vi "getSubscriberInfo.vi"(0 "DeviceName":string="StagingAnalysis", 11 "error in (no error)":errorcluster) -> (4 "DeviceName out":string="StagingAnalysis", 6 "Devices":string[](array[string]), 8 "Alias":string[](array[string]), 10 "Variable header":string[](array[string]), 15 "error out":errorcluster)   [LabVIEW 2011]
panel:
  out "data":string[][](array[string])
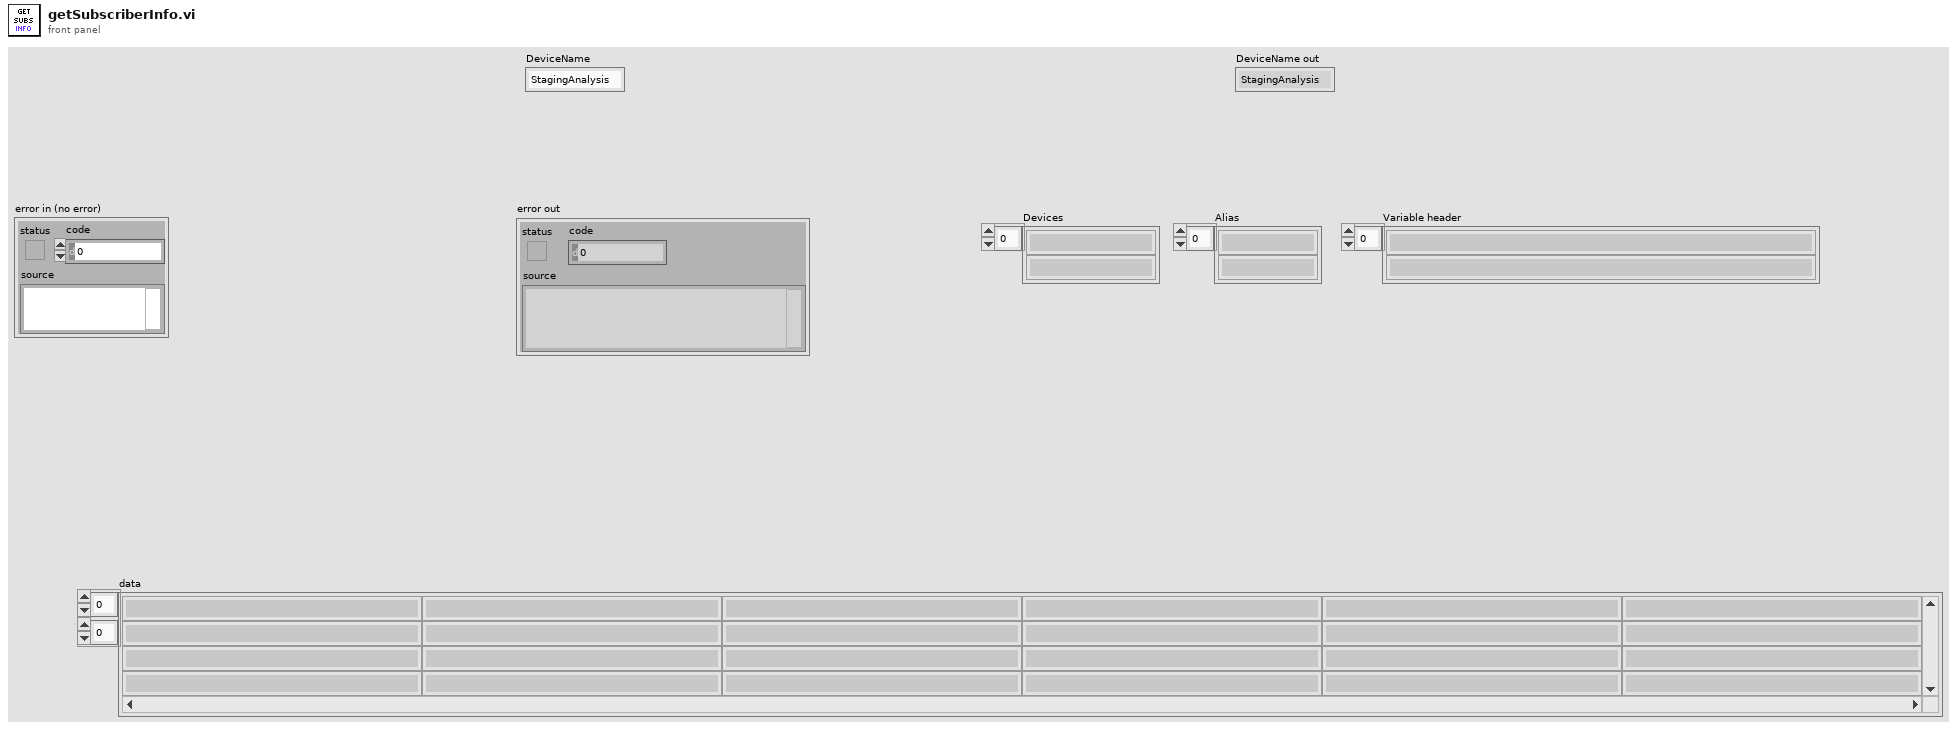
[diagram p1: front panel]
types:
  T1 = typedef "mysql_authentication.ctl" = cluster{"User":string, "Password":string, "Database":string}
  T2 = cluster{"Port":u16, "IP Address":string, "Authentication":T1}
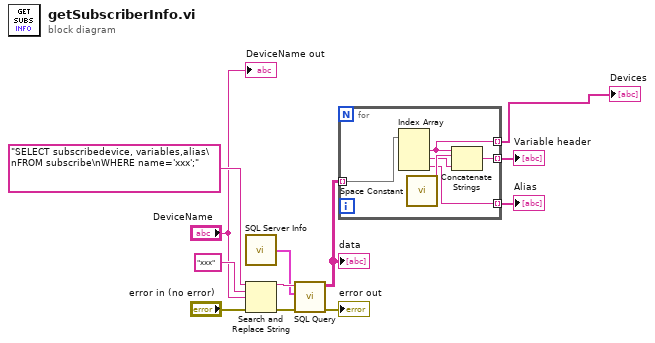
[diagram p0: block diagram]
diagram:
  n1 = call "SQL Server Info.vi"() -> ("SQL Server Info"=w9:T2)
  n2 = Search and Replace String(input string="SELECT subscribedevice, variables,alias\nFROM subscribe\nWHERE name='xxx';", search string="xxx", replace string="DeviceName", error in="error in (no error)") -> (result string=w10:string, error out=w8:errorcluster)  [unwired: 4 in, 2 out]
  n3 = call "SQL Query.vi"("error in (no error)"=w8, "SQL Server Info"=w9, "Query"=w10) -> ("error out"=→"error out":errorcluster, "data"=w6:string[][])  [unwired: 7 in]
  "data" <- w6
  n4 = for {
    tunnel: w6 -> [w18] mode=indexing
    tunnel: [w16] -> w5 mode=indexing
    tunnel: [w15] -> w4 mode=indexing
    tunnel: [w13] -> w1 mode=indexing
    n5 = Index Array(array=w18) -> (element #1=w13:string, element #2=w14:string, element #3=w15:string)  [unwired: 3 in]
    n6 = call "Space Constant.vi"() -> ("String"=w17:string)
    n7 = Concatenate Strings(w13, w17, w14) -> (w16:string)
  }
  "Variable header" <- w5
  "Alias" <- w4
  "Devices" <- w1
  "DeviceName out" <- "DeviceName"
